vi "Data Logging using TDMS.vi"() -> ()   [LabVIEW 2011]
panel:
  out "output row":dbl[](array[numeric])
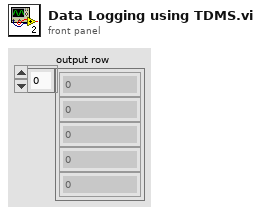
[diagram p1: front panel]
types:
  T1 = enum16{"open", "open or create", "create or replace", "create", "open (read-only)"}
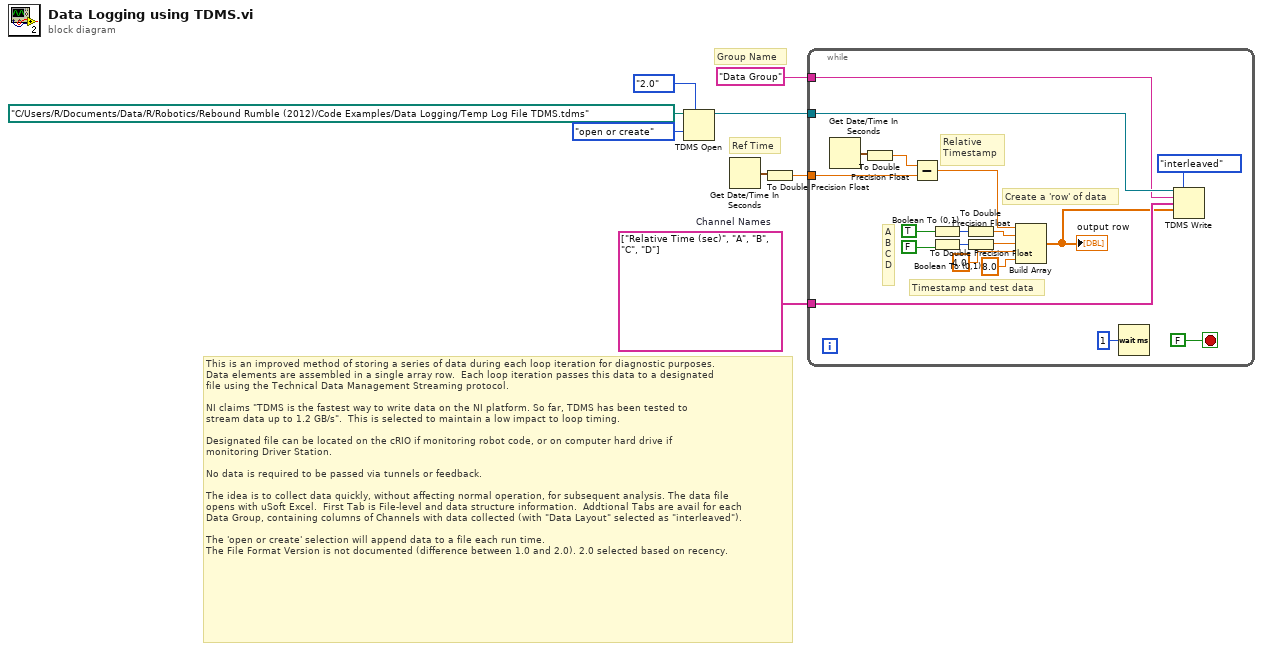
[diagram p0: block diagram]
diagram:
  w2 = string[] ["Relative Time (sec)", "A", "B", "C", "D"]  # Channel Names
  # "Group Name"
  # "Ref Time"
  # "This is an improved method of storing a series of data during each loop iteration for diagnostic purposes.\nData elements are assembled in a single array row.  Each loop iteration passes this data to a designated\nfile using the Technical Data Management Streaming protocol.\n\nNI claims \"TDMS is the fastest way to write data on the NI platform. So far, TDMS has been tested to\nstream data up to 1.2 GB/s\".  This is selected to maintain a low impact to loop timing.\n\nDesignated file can be located on the cRIO if monitoring robot code, or on computer hard drive if \nmonitoring Driver Station.\n\nNo data is required to be passed via tunnels or feedback.\n\nThe idea is to collect data quickly, without affecting normal operation, for subsequent analysis. The data file\nopens with uSoft Excel.  First Tab is File-level and data structure information.  Addtional Tabs are avail for each\nData Group, containing columns of Channels with data collected (with \"Data Layout\" selected as \"interleaved\").\n\nThe 'open or create' selection will append data to a file each run time.\nThe File Format Version is not documented (difference between 1.0 and 2.0). 2.0 selected based on recency."
  n1 = TDMS Open(7:enum16{"1.0", "2.0"}."2.0" ("file format version (2.0)"), 10:T1."open or create" ("operation (0:open)"), 11:path "C:/Users/R/Documents/Data/R/Robotics/Rebound Rumble (2012)/Code Examples/Data Logging/Temp Log File TDMS.tdms" ("file path")) -> (3:w6:refnum<k34>)  [unwired: 3 in, 1 out]
  n2 = Get Date/Time In Seconds() -> (seconds since 1Jan1904=w8:timestamp)
  n3 = To Double Precision Float(number=w8) -> (double precision float=w7:dbl)
  n4 = while {
    tunnel: w7 -> [w23]
    tunnel: w6 -> [w18]
    tunnel: w2 -> [w15]
    tunnel: "Data Group" ("group name in (Untitled)") -> [w17]
    stop <- FALSE stop-if-true
    # "A\nB\nC\nD"
    # "Relative\nTimestamp"
    # "Create a 'row' of data"
    # "Timestamp and test data"
    n5 = Get Date/Time In Seconds() -> (seconds since 1Jan1904=w25:timestamp)
    n6 = To Double Precision Float(number=w25) -> (double precision float=w24:dbl)
    n7 = Subtract(x=w24, y=w23) -> (x-y=w13:dbl)
    n8 = Boolean To (0,1)(Boolean=TRUE) -> (0, 1=w26:i16)
    n9 = Boolean To (0,1)(Boolean=FALSE) -> (0, 1=w27:i16)
    n10 = To Double Precision Float(number=w26) -> (double precision float=w14:dbl)
    n11 = To Double Precision Float(number=w27) -> (double precision float=w12:dbl)
    n12 = Build Array(w13, w14, w12, 4.0 ("element"), 8.0 ("element")) -> (w11:dbl[])
    "output row" <- w11
    n13 = Wait (ms)(milliseconds to wait=u32 1) -> ()  [unwired: 1 out]
    n14 = TDMS Write(0:w18, 1:enum16{"decimated", "interleaved"}."interleaved" ("data layout (0:decimated)"), 5:w17, 7:w15, 9:w11) -> ()  [unwired: 1 in, 4 out]
  }
